vi "Read Grabbed Tool.vi"(8 "error in (no error)":errorcluster, 11 "GrabberTool Class in":refnum<class "GrabberTool Class.lvclass">) -> (0 "error out":errorcluster, 2 "Grabbed Tool":enum16{"Weight Tool", "Stamp Tool", "Nothing"}(ring)=enum."Nothing", 3 "GrabberTool Class out":refnum<class "GrabberTool Class.lvclass">)   [LabVIEW 2011, in "GrabberTool Class.lvclass"]
uses:
  GrabberTool Class.lvclass
  GrabberTool Class.lvclass/GrabberTool Class.ctl
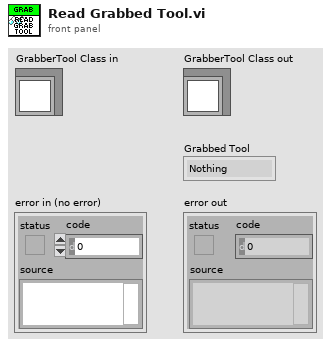
[diagram p1: front panel]
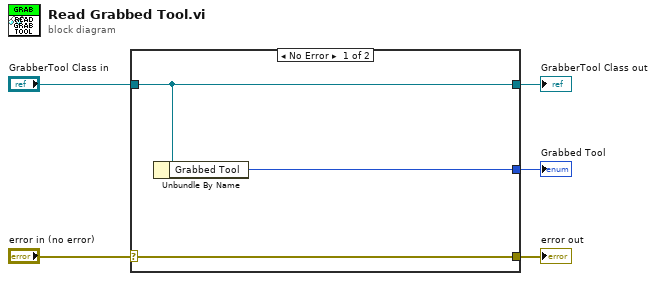
[diagram p0: block diagram]
diagram:
  n1 = case shown="No Error" "error in (no error)" {
    selector: "error in (no error)" -> [w8 w9]
    tunnel: [w8 w9] -> w4
    tunnel: [w7 w10] -> w2
    tunnel: "GrabberTool Class in" -> [w7 w10]
    tunnel: [w6 _] -> w1
    frame No Error {
      n2 = Unbundle By Name(w7) -> ("Grabbed Tool"=w6:enum16{"Weight Tool", "Stamp Tool", "Nothing"})
    }
    frame Error {
    }
  }
  "error out" <- w4
  "GrabberTool Class out" <- w2
  "Grabbed Tool" <- w1
